vi "Read Conversion References.vi"(8 "error in (no error)":errorcluster, 11 "DataContainer in":refnum<class "DataContainer.lvclass">) -> (0 "error out":errorcluster, 2 "Conversion References":refnum<k21>[](array[refnum]), 3 "DataContainer out":refnum<class "DataContainer.lvclass">)   [LabVIEW 2023, in "DataContainer.lvclass"]
uses:
  DataContainer.lvclass
  DataContainer.lvclass/DataContainer.ctl
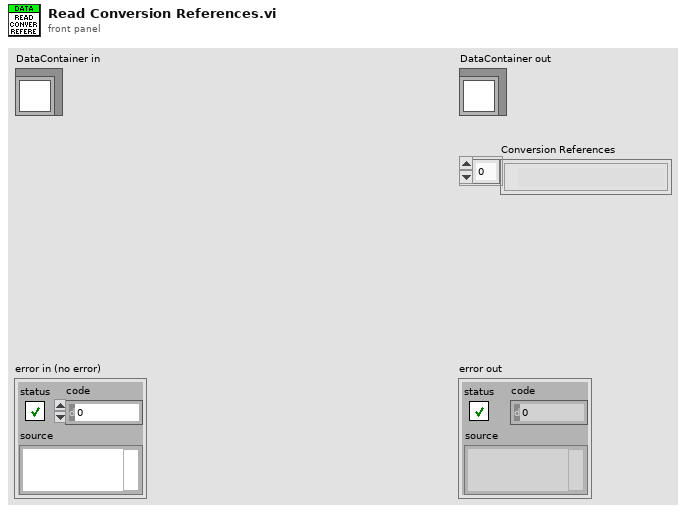
[diagram p1: front panel]
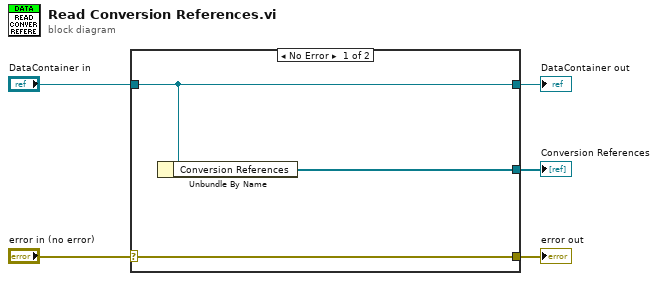
[diagram p0: block diagram]
diagram:
  n1 = case shown="No Error" "error in (no error)" {
    selector: "error in (no error)" -> [w8 w9]
    tunnel: [w8 w9] -> w4
    tunnel: [w7 w10] -> w2
    tunnel: "DataContainer in" -> [w7 w10]
    tunnel: [w6 _] -> w1
    frame No Error {
      n2 = Unbundle By Name(w7) -> ("Conversion References"=w6:refnum<k21>[])
    }
    frame Error {
    }
  }
  "error out" <- w4
  "DataContainer out" <- w2
  "Conversion References" <- w1
